vi "Read FW Version.vi"(8 "errorIN":errorcluster, 11 "LCD in":refnum<class "LCD Retarder.lvclass">) -> (0 "error out":errorcluster, 1 "FW Version":dbl, 3 "LCD out":refnum<class "LCD Retarder.lvclass">)   [LabVIEW 2023, in "LCD Retarder.lvclass"]
uses:
  LCD Retarder.lvclass
  LCD Retarder.lvclass/LCD Retarder.ctl
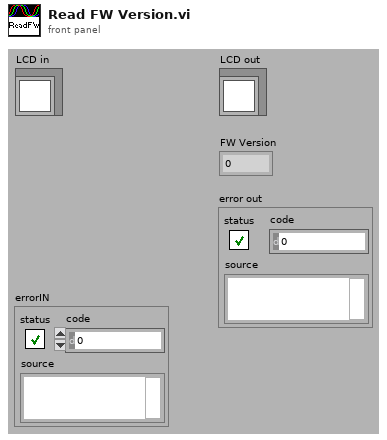
[diagram p1: front panel]
types:
  T1 = cluster{"Device Handle":u32, "Pipe 0 Handle":u32, "Pipe 1 Handle":u32}
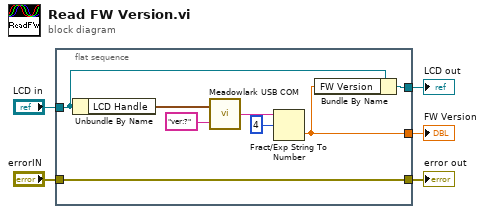
[diagram p0: block diagram]
diagram:
  n1 = flat-sequence {
    tunnel: [w6] -> w1
    tunnel: [w7] -> w2
    tunnel: "LCD in" -> [w9]
    tunnel: "errorIN" -> [w10]
    tunnel: [w10] -> w5
    frame #0 {
      n2 = Unbundle By Name(w9) -> ("LCD Handle"=w8:T1)
      n3 = call "Meadowlark USB COM.vi"("WRITE IN String"="ver:?", "USB Open Device Cluster"=w8) -> ("READ OUT String"=w11:string)
      n4 = Fract/Exp String To Number(string=w11, offset=4) -> (number=w6:dbl)  [unwired: 3 out]
      n5 = Bundle By Name(cluster=w9, "FW Version"=w6) -> (w7:refnum<class "LCD Retarder.lvclass">)
    }
  }
  "error out" <- w5
  "LCD out" <- w2
  "FW Version" <- w1
